vi "Test Insert, Jig Refereneced.vi"() -> ()   [LabVIEW 2013]
uses:
  <vilib>/Analysis/Matrix/Datatypes/RealMatrix.ctl
  Arm Globals.vi
  Move/Move Axis.vi
  ROS/Code/Console/Servers/ServerSubs/(nist) Arm Globals.vi
  ROS/Code/SubVIs/BaxterSide.ctl
  <vilib>/Analysis/Matrix/NI_Matrix.lvlib
panel:
  out "Object Current":T1 format="%.3f"
  out "R:Joints Pose":T1 format="%.3f"
  out "y":dbl
  out "x":dbl
  out "Converted":dbl[](array[numeric]) format="%.3f"
  out "Direct":dbl[](array[numeric]) format="%.3f"
  out "R:Joints":dbl[](array[numeric])=[-0.416, -0.52, 1.12, -3.856, -0.084, -0.176, 0.14]
  out "Joints":dbl[](array[numeric])
  in  "Stop":bool
  out "Status":string
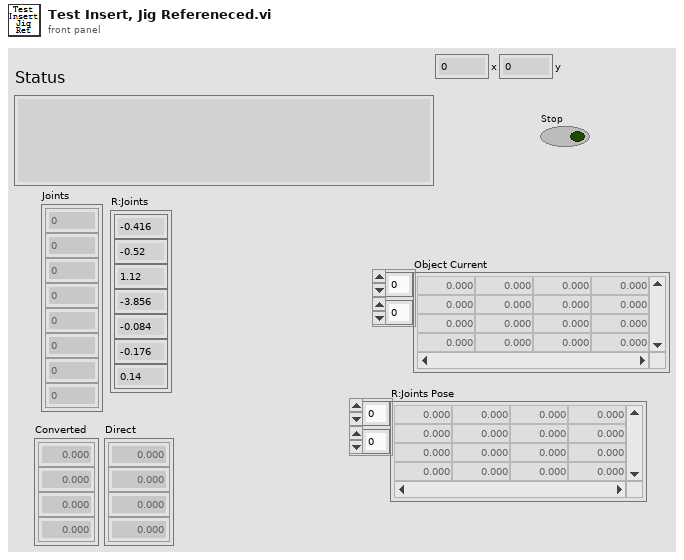
[diagram p1: front panel]
types:
  T1 = typedef "NI_Matrix.lvlib/RealMatrix.ctl" = dbl[][]
  T2 = cluster{"X":dbl, "Y":dbl, "Z":dbl, "O":dbl, "A":dbl, "T":dbl}
  T3 = typedef "BaxterSide.ctl" = enum16{"left", "right"}
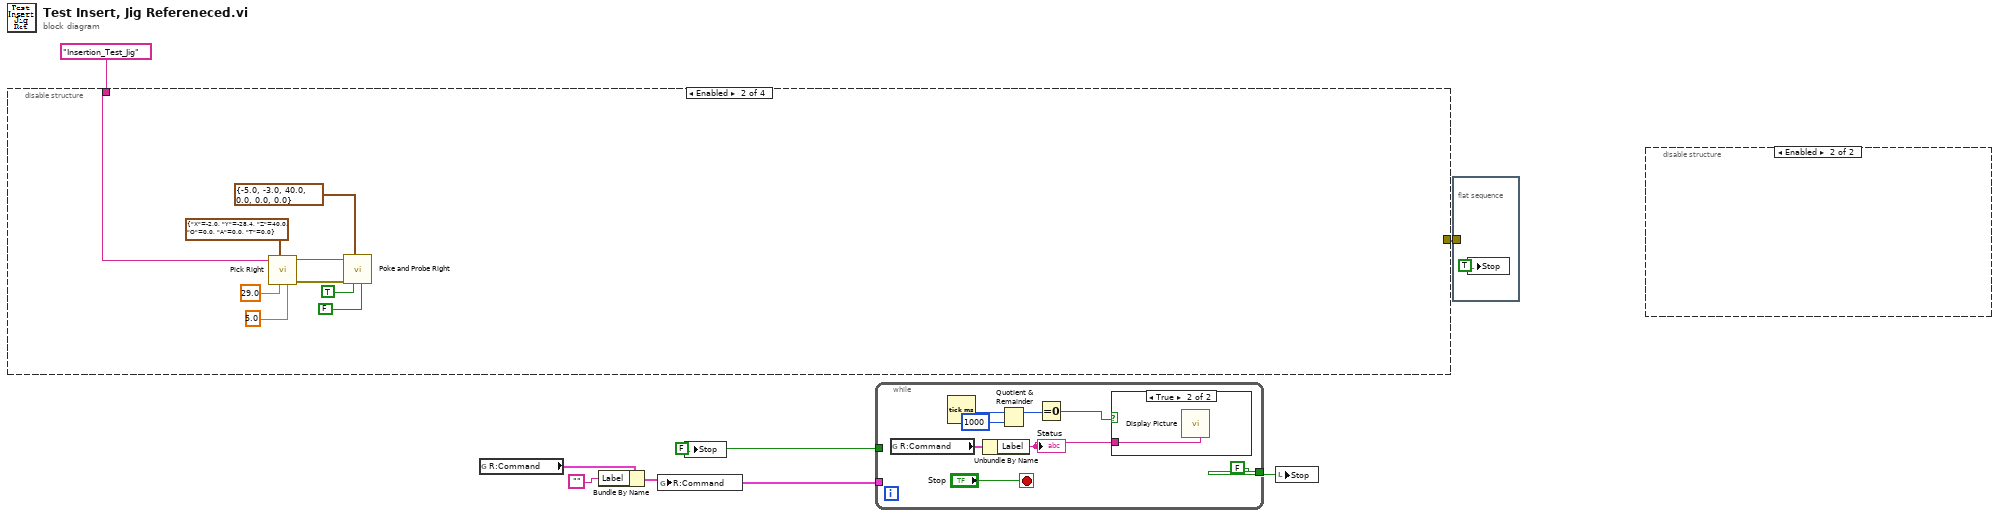
[diagram p0: block diagram]
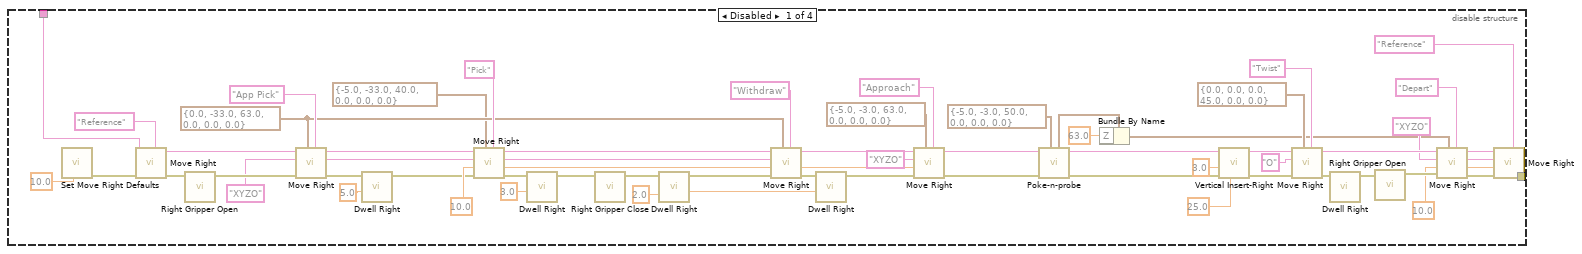
[diagram p2: hidden frame]
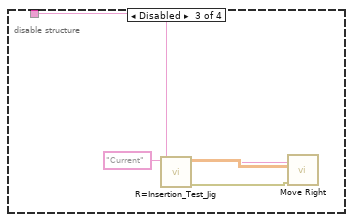
[diagram p3: hidden frame]
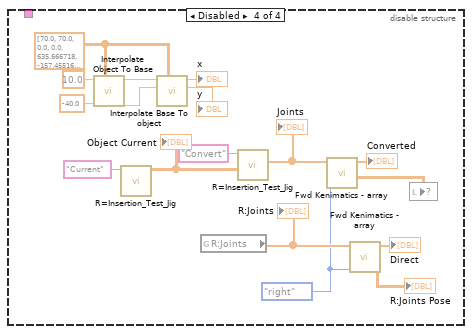
[diagram p4: hidden frame]
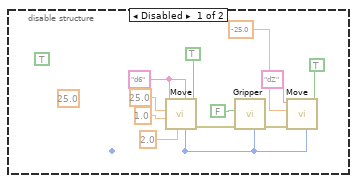
[diagram p5: hidden frame]
diagram:
  w2 = FALSE ("Stop")
  n1 = disable-structure shown="Enabled" {
    disable-tunnel: [w68 _ _ _] -> w4
    disable-tunnel: "Insertion_Test_Jig" ("Location") -> [w31 w78 w79 _]
    frame Disabled {
      w19 = 2.0 ("Wait Time")
      w24 = "XYZO" ("Mask")
      w29 = T2 {"X"=0.0, "Y"=-33.0, "Z"=63.0, "O"=0.0, "A"=0.0, "T"=0.0} ("Goal Axes")
      n2 = call "Set Move Right Defaults.vi"("Speed"=10.0) -> ("error out"=w45:errorcluster)  [unwired: 10 in]
      n3 = call "Move Right.vi"("Label"="Reference", "error in"=w45, "Location"=w31) -> ("error out"=w44:errorcluster, "Location Out"=w56:string)  [unwired: 4 in, 3 out]
      n4 = call "Right Gripper Open.vi"("error in"=w44) -> ("error out"=w43:errorcluster)  [unwired: 10 in]
      n5 = call "Move Right.vi"("Label"="App Pick", "Goal"=w29, "error in"=w43, "Mask"=w24, "Location"=w56) -> ("error out"=w42:errorcluster, "Location Out"=w55:string)  [unwired: 2 in, 3 out]
      n6 = call "Dwell Right.vi"("Wait Time"=5.0 ("Wait (s)"), "error in"=w42) -> ("error out"=w8:errorcluster)  [unwired: 9 in]
      n7 = call "Move Right.vi"("Label"="Pick", "Goal"=T2 {"X"=-5.0, "Y"=-33.0, "Z"=40.0, "O"=0.0, "A"=0.0, "T"=0.0} ("Goal Axes"), "error in"=w8, "Speed"=10.0, "Mask"=w24, "Location"=w55) -> ("error out"=w26:errorcluster, "Speed Out"=w22:dbl, "Mask Out"=w25:string, "Location Out"=w27:string)  [unwired: 1 in, 1 out]
      n8 = call "Dwell Right.vi"("Wait Time"=3.0, "error in"=w26) -> ("error out"=w10:errorcluster)  [unwired: 9 in]
      n9 = call "Right Gripper Close.vi"("error in"=w10) -> ("error out"=w30:errorcluster)  [unwired: 9 in, 1 out]
      n10 = call "Dwell Right.vi"("Wait Time"=w19, "error in"=w30) -> ("error out"=w9:errorcluster)  [unwired: 9 in]
      n11 = call "Move Right.vi"("Label"="Withdraw", "Goal"=w29, "error in"=w9, "Speed"=w22, "Mask"=w25, "Location"=w27) -> ("error out"=w37:errorcluster, "Speed Out"=w23:dbl, "Location Out"=w53:string)  [unwired: 1 in, 2 out]
      n12 = call "Dwell Right.vi"("Wait Time"=w19, "error in"=w37) -> ("error out"=w36:errorcluster)  [unwired: 9 in]
      n13 = call "Move Right.vi"("Label"="Approach", "Goal"=T2 {"X"=-5.0, "Y"=-3.0, "Z"=63.0, "O"=0.0, "A"=0.0, "T"=0.0} ("Goal Axes"), "error in"=w36, "Speed"=w23, "Mask"="XYZO", "Location"=w53) -> ("error out"=w17:errorcluster, "Location Out"=w18:string)  [unwired: 1 in, 3 out]
      n14 = call "Poke-n-probe.vi"("Goal"=T2 {"X"=-5.0, "Y"=-3.0, "Z"=50.0, "O"=0.0, "A"=0.0, "T"=0.0} ("Goal Axes"), "error in"=w17, "Location"=w18) -> ("error out"=w16:errorcluster, "Location Out"=w15:string, "Pose"=w11:T2)  [unwired: 4 in, 2 out]
      n15 = Bundle By Name(cluster=w11, "Z"=63.0 ("X")) -> (w12:T2)
      n16 = call "Vertical Insert-Right.vi"("depth"=25.0, "error in"=w16, "Speed"=3.0, "Location"=w15) -> ("error out"=w40:errorcluster, "Location Out"=w32:string)  [unwired: 6 in]
      n17 = call "Move Right.vi"("Label"="Twist", "Goal"=T2 {"X"=0.0, "Y"=0.0, "Z"=0.0, "O"=45.0, "A"=0.0, "T"=0.0} ("Goal Axes"), "error in"=w40, "Mask"="O", "Location"=w32) -> ("error out"=w39:errorcluster, "Location Out"=w52:string)  [unwired: 2 in, 3 out]
      n18 = call "Dwell Right.vi"("error in"=w39) -> ("error out"=w35:errorcluster)  [unwired: 10 in]
      n19 = call "Right Gripper Open.vi"("error in"=w35) -> ("error out"=w38:errorcluster)  [unwired: 10 in]
      n20 = call "Move Right.vi"("Label"="Depart", "Goal"=w12, "error in"=w38, "Speed"=10.0, "Mask"="XYZO", "Location"=w52) -> ("error out"=w62:errorcluster, "Speed Out"=w54:dbl, "Mask Out"=w46:string, "Location Out"=w51:string)  [unwired: 1 in, 1 out]
      n21 = call "Move Right.vi"("Label"="Reference", "error in"=w62, "Speed"=w54, "Mask"=w46, "Location"=w51) -> ("error out"=w68:errorcluster)  [unwired: 2 in, 4 out]
    }
    frame Enabled {
      n22 = call "Pick Right.vi"("Threshold"=sgl 5.0, "Target Position"=sgl 29.0, "Pick"=T2 {"X"=-2.0, "Y"=-28.4, "Z"=40.0, "O"=0.0, "A"=0.0, "T"=0.0}, "Location"=w78) -> ("error out"=w73:errorcluster, "Location Out"=w74:string)  [unwired: 6 in]
      n23 = call "Poke and Probe Right.vi"("Tap In?"=FALSE, "Release Part"=TRUE, "Goal"=T2 {"X"=-5.0, "Y"=-3.0, "Z"=40.0, "O"=0.0, "A"=0.0, "T"=0.0}, "error in"=w73, "Location"=w74) -> ()  [unwired: 4 in, 3 out]
    }
    frame Disabled {
      n24 = call "R=Insertion_Test_Jig.vi"("Command"="Current") -> ("error out"=w80:errorcluster, "Pose Out"=w81:T1)  [unwired: 8 in, 1 out]
      n25 = call "Move Right.vi"("Goal"=w79, "error in"=w80, "Mask"=w81) -> ()  [unwired: 4 in, 5 out]
    }
    frame Disabled {
      w87 = dbl[][] [[70.0, 70.0, 0.0, 0.0, 635.666718, -157.45516, -50.0, -2.259266], [70.0, -70.0, 0.0, 0.0, 633.682949, -298.606674, -50.0, -2.79925], [-70.0, 70.0, 0.0, 0.0, 501.946047, -154.501775, -50.0, -3.895959], [-70.0, -70.0, 0.0, 0.0, 494.372979, -294.486847, -50.0, -3.439588]] ("Table")
      w95 = BaxterSide."right" ("Side")
      n26 = call "Interpolate Object To Base.vi"("Table"=w87, "Y"=-40.0, "X"=10.0) -> ("y"=w90:dbl, "x"=w91:dbl)  [unwired: 5 in, 2 out]
      n27 = call "R=Insertion_Test_Jig.vi"("Command"="Current") -> ("Pose Out"=w97:T1)  [unwired: 8 in, 2 out]
      "Object Current" <- w97
      n28 = call "Interpolate Base To object.vi"("Table"=w87, "Y"=w90, "X"=w91) -> ("y"=→"y":dbl, "x"=→"x":dbl)  [unwired: 5 in, 2 out]
      n29 = global read "(nist) Arm Globals.vi" "R:Joints"() -> (w96:dbl[])
      "R:Joints" <- w96
      n30 = call "R=Insertion_Test_Jig.vi"("Matrix"=w97, "Command"="Convert") -> ("Joints"=w94:dbl[])  [unwired: 7 in, 2 out]
      "Joints" <- w94
      n31 = call "Fwd Kenimatics - array.vi"("Side"=w95, "Joints"=w94) -> ("Matrix"=w84:T1, "Position"=→"Converted":dbl[])  [unwired: 8 in]
      n32 = call "Fwd Kenimatics - array.vi"("Side"=w95, "Joints"=w96) -> ("Matrix"=→"R:Joints Pose":T1, "Position"=→"Direct":dbl[])  [unwired: 8 in]
      n33 = local write item#-1(w84) -> ()
    }
  }
  n34 = global read "Arm Globals.vi" "R:Command"() -> (w7:cluster{"Label":string, "Angles":dbl[]})
  n35 = Bundle By Name(cluster=w7, "Label"="") -> (w5:cluster{"Label":string, "Angles":dbl[]})
  n36 = global write "Arm Globals.vi" "R:Command"(w5) -> ()
  n37 = local write "Stop"(w2) -> ()
  n38 = while {
    tunnel: w5 -> [_]
    tunnel: [FALSE] -> w3
    tunnel: w2 -> [_]
    stop <- "Stop" stop-if-true
    n39 = global read "Arm Globals.vi" "R:Command"() -> (w107:cluster{"Label":string, "Angles":dbl[]})
    n40 = Tick Count (ms)() -> (millisecond timer value=w104:u32)
    n41 = Unbundle By Name(w107) -> ("Label"=w100:string)
    "Status" <- w100
    n42 = Quotient & Remainder(x=w104, y=u32 1000) -> (x-y*floor(x/y)=w102:u32)  [unwired: 1 out]
    n43 = Equal To 0?(x=w102) -> (x = 0?=w101:bool)
    n44 = case shown="True" w101 {
      tunnel: w100 -> [_ w108]
      frame False {
      }
      frame True {
        n45 = call "Display Picture.vi"("Comment"=w108) -> ()  [unwired: 10 in, 1 out]
      }
    }
  }
  n46 = local write "Stop"(w3) -> ()
  n47 = flat-sequence {
    tunnel: w4 -> [_]
    frame #0 {
      n48 = local write "Stop"(TRUE ("Stop")) -> ()
    }
  }
  n49 = disable-structure shown="Enabled" {
    frame Disabled {
      (unwired) 25.0 ("depth")
      w118 = "d6" ("Location")
      w122 = TRUE ("Make Vertical")
      n50 = call-poly "Move.vi"("Make Vertical"=TRUE, "Side"=w110, "Label"=w118, "Wait Time"=2.0, "Speed"=1.0, "Value"=25.0 ("depth"), "Location"=w118) -> ("error out"=w119:errorcluster, "error in"=w120:errorcluster)  [unwired: 3 in]
      n51 = call "Gripper.vi"("error in"=w119, "Open?"=FALSE) -> ("error out"=w114:errorcluster, "Side"=w110:T3)  [unwired: 7 in, 1 out]
      n52 = call-poly "Move.vi"("Make Vertical"=TRUE, "Side"=w110, "error in"=w114, "Value"=-25.0 ("Speed (mm/s)"), "Location"="dZ") -> ()  [unwired: 6 in, 1 out]
    }
    frame Enabled {
    }
  }
